vi "EIP PLC Info.vi"(6 "Path":string, 7 "Timeout":i32) -> (1 "Device Settings":T1)   [LabVIEW 2011, in "Ethernet IP Custom Device Custom Device.lvlib"]
doc: "VI that creates a cluster including the timeout when communicating with Ethernet/IP + the actual network path to the PLC."
uses:
  Ethernet IP Custom Device Custom Device.lvlib
  EIP Device Settings.ctl
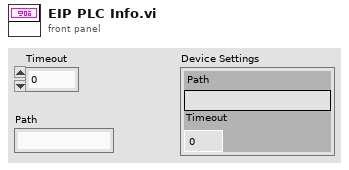
[diagram p1: front panel]
types:
  T1 = typedef "Ethernet IP Custom Device Custom Device.lvlib/EIP Device Settings.ctl" = cluster{"Path":string, "Timeout":i32}
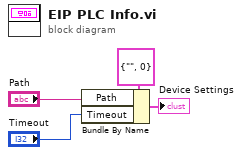
[diagram p0: block diagram]
diagram:
  n1 = Bundle By Name(cluster=T1 {"Path"="", "Timeout"=0} ("Device Settings"), "Path"="Path", "Timeout"="Timeout") -> (→"Device Settings":T1)
